vi "ReadChildren.vi"(8 "error in":errorcluster, 11 "node in":refnum<class "NISE_CEF_Node.lvclass">) -> (0 "error out":errorcluster, 2 "output array":T1[](array[typedef]), 3 "node out":refnum<class "NISE_CEF_Node.lvclass">)   [LabVIEW 2013, in "NISE_CEF_Node.lvclass"]
uses:
  NISE_CEF_Node.lvclass
  NodeRef.ctl
  NISE_CEF_Node.lvclass/NISE_CEF_Node.ctl
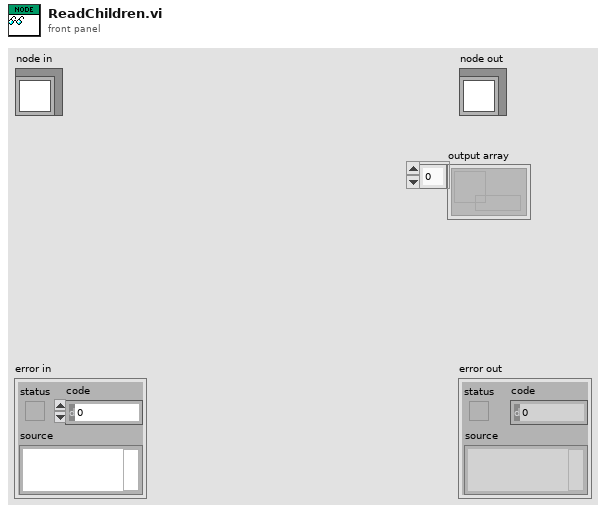
[diagram p1: front panel]
types:
  T1 = typedef "NISE_CEF_Node.lvclass/NodeRef.ctl" = refnum<data-value>
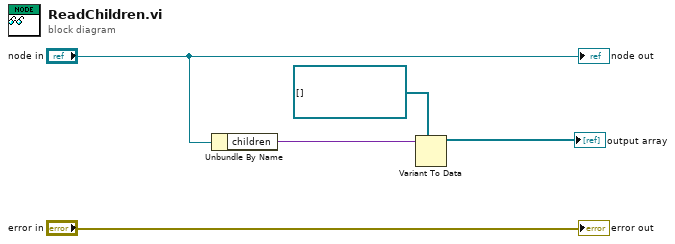
[diagram p0: block diagram]
diagram:
  n1 = Unbundle By Name("node in") -> ("children"=w3:variant)
  n2 = Variant To Data(type=refnum<data-value>[] [], Variant=w3) -> (data=→"output array":refnum<data-value>[])  [unwired: 1 in, 1 out]
  "error out" <- "error in"
  "node out" <- "node in"
